vi "Items to Names.vi"(7 "Items":T1(array[cluster])) -> (3 "Names":string[](array[string]))   [LabVIEW 2019, in "Selector.lvclass"]
uses:
  Selector.lvclass
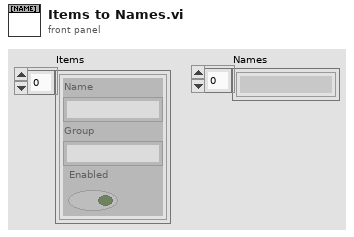
[diagram p1: front panel]
types:
  T1 = cluster{"Name":string, "Group":string, "Enabled":bool}[]
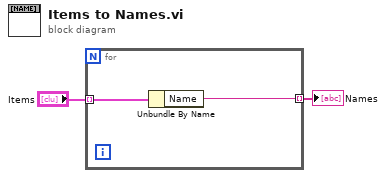
[diagram p0: block diagram]
diagram:
  n1 = for {
    tunnel: "Items" -> [w4] mode=indexing
    tunnel: [w3] -> w1 mode=indexing
    n2 = Unbundle By Name(w4) -> ("Name"=w3:string)
  }
  "Names" <- w1
